vi "SNMP Parse SNMP Packet.vi"(9 "SNMP Packet":u8[](array[numeric]) format="%.0x") -> (0 "SnmpData":string[][](array[string]), 1 "Error Index":i32, 2 "Error Status String":string, 3 "Error Status":i32, 4 "Req ID":i32, 5 "Community String":string, 7 "SNMP version":i32)   [LabVIEW 2017]
doc: "This VI parses a SNMP packet and returns the pertitent SNMP header information and the SNMP data."
uses:
  CTL - SNMP Types.ctl
panel:
  in  "SNMP Data Types":T1={"Integer"=2, "Octet-String"=4, "NULL"=5, "Object Identifier"=6, "Sequence"=48, "IP Address"=64, "Counter"=65, "Gauge"=66, "TimeTicks"=67, "Opaque"=68, "GetRequest-PDU"=160, "GetNextRequest-PDU"=161, "GetResponse-PDU"=162, "SetRequest-PDU"=163, "Trap-PDU"=164} {"Opaque" format="%.0x"; "TimeTicks" format="%.0x"; "Gauge" format="%.0x"; "Counter" format="%.0x"; "IP Address" format="%.0x"; "NULL" format="%.0x"; "Trap-PDU" format="%.0x"; "SetRequest-PDU" format="%.0x"; "GetNextRequest-PDU" format="%.0x"; "Object Identifier" format="%.0x"; "Sequence" format="%.0x"; "GetResponse-PDU" format="%.0x"; "GetRequest-PDU" format="%.0x"; "Octet-String" format="%.0x"; "Integer" format="%.0x"}
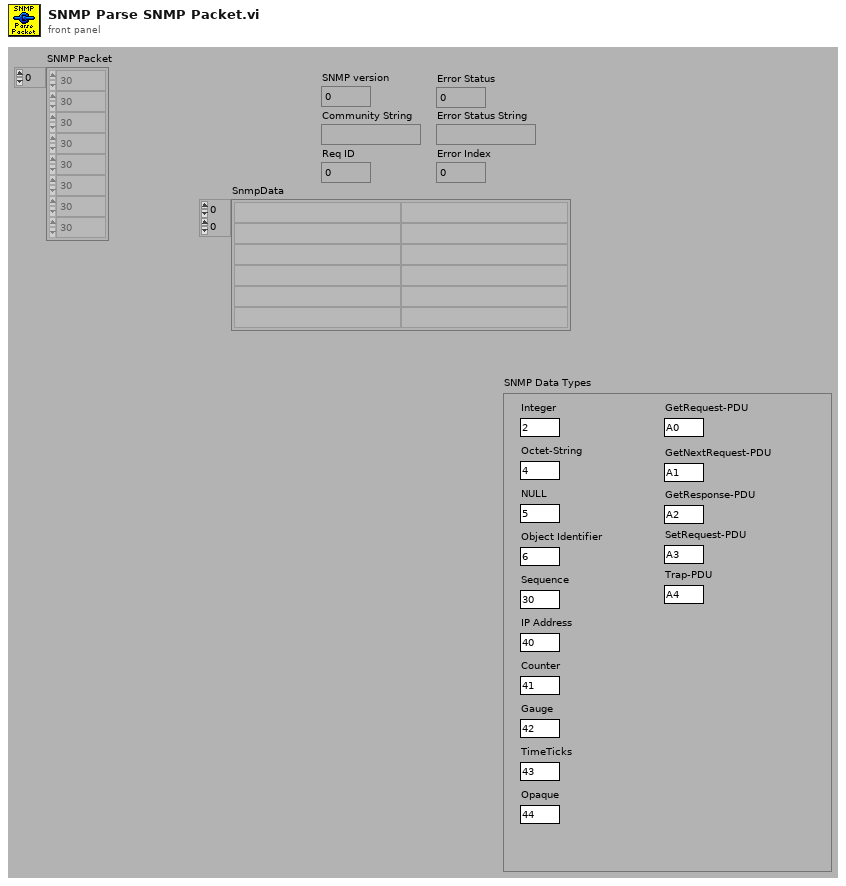
[diagram p1: front panel]
types:
  T1 = typedef "CTL - SNMP Types.ctl" = cluster{"Integer":u8, "Octet-String":u8, "NULL":u8, "Object Identifier":u8, "Sequence":u8, "IP Address":u8, "Counter":u8, "Gauge":u8, "TimeTicks":u8, "Opaque":u8, "GetRequest-PDU":u8, "GetNextRequest-PDU":u8, "GetResponse-PDU":u8, "SetRequest-PDU":u8, "Trap-PDU":u8}
  T2 = cluster{"Numeric":u32, "Octet String":string, "Byte Array":u8[]}
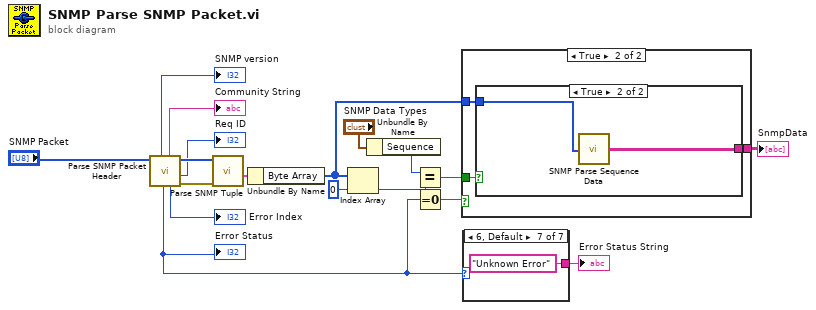
[diagram p0: block diagram]
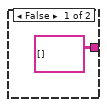
[diagram p2: hidden frame]
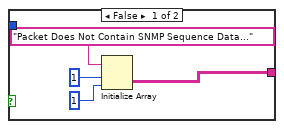
[diagram p3: hidden frame]
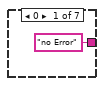
[diagram p4: hidden frame]
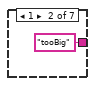
[diagram p5: hidden frame]
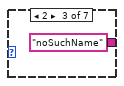
[diagram p6: hidden frame]
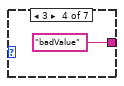
[diagram p7: hidden frame]
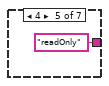
[diagram p8: hidden frame]
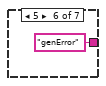
[diagram p9: hidden frame]
diagram:
  n1 = call "Parse SNMP Packet Header.vi"("SNMP Packet"="SNMP Packet") -> ("error out"=w18:errorcluster, "Req ID"=→"Req ID":i32, "SNMP Packet Out"=w4:u8[], "Error Index"=→"Error Index":i32, "Community String"=→"Community String":string, "Error Status"=w6:i32, "SNMP version"=→"SNMP version":i32)  [unwired: 2 in, 2 out]
  "Error Status" <- w6
  n2 = call "Parse SNMP Tuple.vi"("error in (no error)"=w18, "SNMP Packet In"=w4) -> ("Data Out"=w17:T2)  [unwired: 9 out]
  n3 = Unbundle By Name(w17) -> ("Byte Array"=w11:u8[])
  n4 = Index Array(array=w11, index=0 ("Index")) -> (element=w15:u8)
  n5 = Unbundle By Name("SNMP Data Types") -> ("Sequence"=w14:u8)
  n6 = Equal?(x=w14, y=w15) -> (x = y?=w12:bool)
  n7 = Equal To 0?(x=w6) -> (x = 0?=w7:bool)
  n8 = case shown="True" w7 {
    tunnel: [string[][] [] ("SequenceAsStrings") w22] -> w13
    tunnel: w12 -> [_ w21]
    tunnel: w11 -> [_ w20]
    frame False {
    }
    frame True {
      n9 = case shown="True" w21 {
        tunnel: [w23 w28] -> w22
        tunnel: w20 -> [_ w27]
        frame False {
          n10 = Initialize Array("Packet Does Not Contain SNMP Sequence Data...", 1, 1) -> (w23:string[][])
        }
        frame True {
          n11 = call "SNMP Parse Sequence Data.vi"("Sequence Data"=w27) -> ("SequenceAsStrings"=w28:string[][])
        }
      }
    }
  }
  "SnmpData" <- w13
  n12 = case shown="6, Default" w6 {
    tunnel: ["no Error" "tooBig" "noSuchName" "badValue" "readOnly" "genError" "Unknown Error"] -> w9
    frame 0 {
    }
    frame 1 {
    }
    frame 2 {
    }
    frame 3 {
    }
    frame 4 {
    }
    frame 5 {
    }
    frame 6, Default {
    }
  }
  "Error Status String" <- w9
